vi "Point to End of Log File.vi"(8 "error in (no error)":errorcluster, 11 "Byte Stream File in":refnum<file>) -> (0 "error out":errorcluster, 3 "Byte Stream File out":refnum<file>)   [LabVIEW 2015, in "Generic Module Library.lvlib" / "Template G_Module.lvlib"]
uses:
  Template G_Module.lvlib
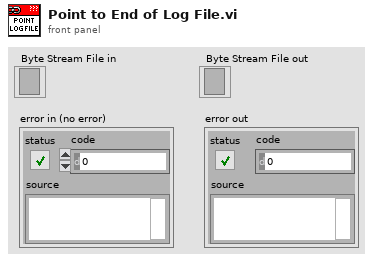
[diagram p1: front panel]
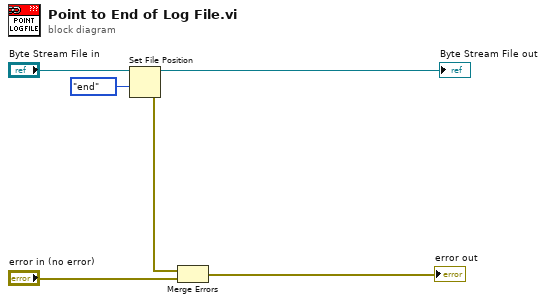
[diagram p0: block diagram]
diagram:
  n1 = Set File Position(refnum="Byte Stream File in", from (0:start)=enum16{"start", "end", "current"}."end") -> (refnum out=→"Byte Stream File out":refnum<file>, error out=w3:errorcluster)  [unwired: 2 in]
  n2 = Merge Errors(w3, "error in (no error)") -> (→"error out":errorcluster)
